vi "mecanum tank 1 sl.vi"   [LabVIEW 2012, in "Mecanum Drive.lvrbt"]
uses:
  Mecanum Drive.lvrbt
  <vilib>/NXT/Hardware/Plugins/Tetrix DC Motor/TetrixDCMotorAddress.ctl
  <vilib>/NXT/NXTIO Xnodes/NXTIONodeSubVIs/TETRIX IO Move DC Motors.vi
  <vilib>/NXT/Dual Mode Library/Display/drawNumber.vi
  <vilib>/NXT/NXTIO Xnodes/NXTIONodeSubVIs/TETRIX IO Check Battery.vi
  <vilib>/NXT/NXTIO Xnodes/NXTIONodeSubVIs/TETRIX IO Stop DC Motors.vi
  <vilib>/NXT/NXTIO Xnodes/AddressXNode/NXTIOAddress.xnode
  <vilib>/NXT/Subs/LVHSConnector.ctl
  <vilib>/NXT/NXTIO Xnodes/NXTIOXNode/NXTIO.xnode
  <vilib>/NXT/LegoClasses/BrickReference/BrickReference.lvclass
panel:
  # "This VI was generated based on your configuration in the Remote Control Editor. You may modify the code as needed for your robot. To test this program for an FTC match, return to the Remote Control Editor, select the \"Run Program\" tab, and choose \"Teleop\"."
types:
  T1 = typedef "TetrixDCMotorAddress.ctl" = i32
  T2 = cluster{"TetrixDCMotor":T1, "TetrixDCMotor 2":T1}
  T3 = typedef "LVHSConnector.ctl" = refnum<class "BrickReference.lvclass">
  T4 = typedef "FTC ControllerState.ctl" = cluster{"Left X":i8, "Left Y":i8, "Right X":i8, "Right Y":i8, "Button Encoding 9-12":u8, "Button Encoding 1-8":u8, "POV":T5}
  T5 = typedef "FTC POVState.ctl" = i8
  T6 = typedef "FTC ButtonEventType.ctl" = enum16{"Pressed", "Released"}
  T7 = cluster{"Button ID":enum16{"None", "Button 1", "Button 2", "Button 3", "Button 4", "Button 5", "Button 6", "Button 7", "Button 8", "Button 9", "Button 10", "Button 11", "Button 12", "POV Up", "POV Up Right", "POV Right", "POV Down Right", "POV Down", "POV Down Left", "POV Left", "POV Up Left"}, "Event Type":T6}[]
  T8 = typedef "FTC ButtonState.ctl" = cluster{"Button 1":bool, "Button 2":bool, "Button 3":bool, "Button 4":bool, "Button 5":bool, "Button 6":bool, "Button 7":bool, "Button 8":bool, "Button 9":bool, "Button 10":bool, "Button 11":bool, "Button 12":bool, "POV":T5}
  T9 = enum16{"None", "Button 1", "Button 2", "Button 3", "Button 4", "Button 5", "Button 6", "Button 7", "Button 8", "Button 9", "Button 10", "Button 11", "Button 12", "POV Up", "POV Up Right", "POV Right", "POV Down Right", "POV Down", "POV Down Left", "POV Left", "POV Up Left"}
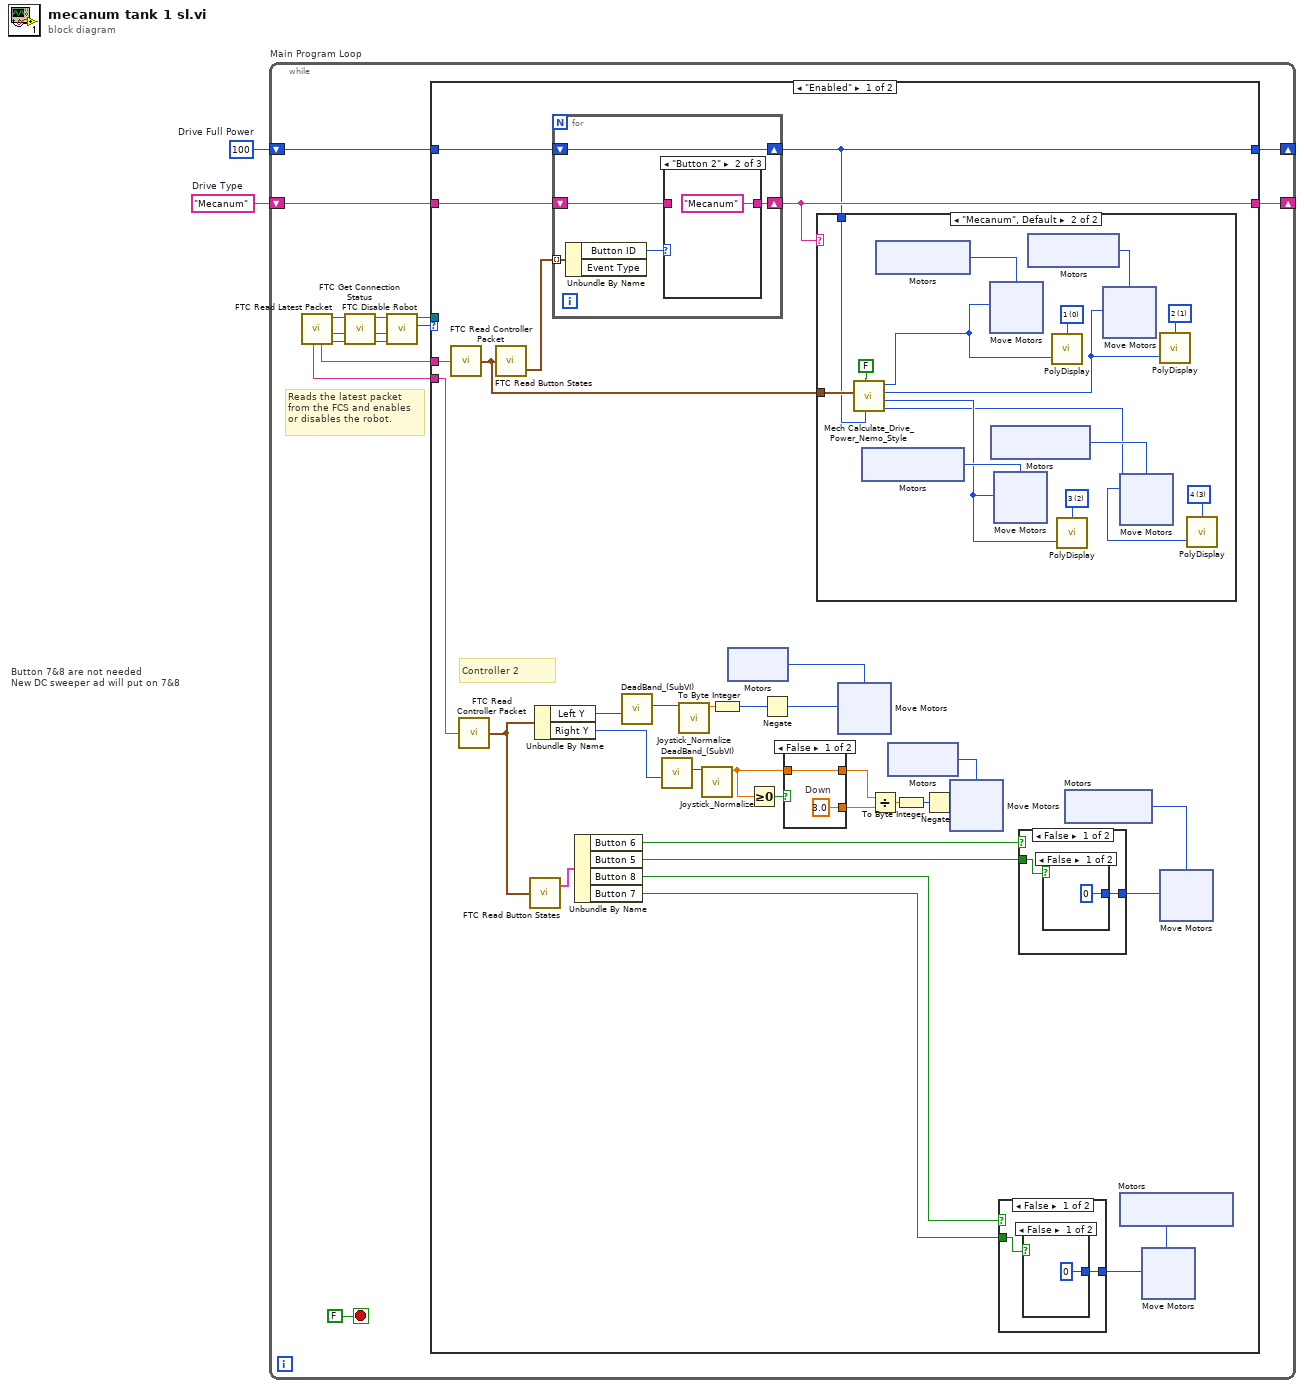
[diagram p0: block diagram]
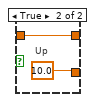
[diagram p2: hidden frame]
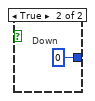
[diagram p3: hidden frame]
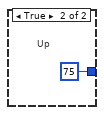
[diagram p4: hidden frame]
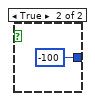
[diagram p5: hidden frame]
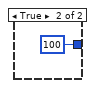
[diagram p6: hidden frame]
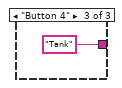
[diagram p9: hidden frame]
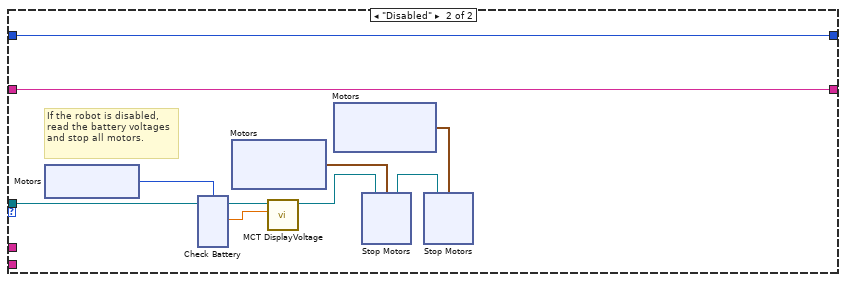
[diagram p10: hidden frame]
diagram:
  w1 = 100  # Drive Full Power
  w2 = "Mecanum"  # Drive Type
  # "Button 7&8 are not needed\nNew DC sweeper ad will put on 7&8"
  n1 = while "Main Program Loop" {
    shift-right: [w5] -> _
    shift-left: w2 -> [w6]
    shift-right: [w3] -> _
    shift-left: w1 -> [w4]
    stop <- FALSE stop-if-true
    # "Reads the latest packet\nfrom the FCS and enables\nor disables the robot."
    n2 = call <vilib>:"FTC Read Latest Packet.vi"() -> ("Packet Received?"=w14:bool, "Stopped?"=w11:bool, "NXT"=w13:T3, "Controller 1"=w16:string, "Controller 2"=w15:string)  [unwired: 6 in, 1 out]
    n3 = call <vilib>:"FTC Get Connection Status.vi"("Packet Received?"=w14, "Stopped?"=w11, "NXT"=w13) -> ("Online?"=w8:bool, "Stopped?"=w9:bool, "NXT"=w10:T3)  [unwired: 5 in]
    n4 = call <vilib>:"FTC Disable Robot.vi"("Online?"=w8, "Stopped?"=w9, "NXT"=w10) -> ("Enabled?"=w12:enum16{"Disabled", "Enabled"}, "NXT"=w7:T3)  [unwired: 3 in]
    n5 = case "disableCase" shown="\"Enabled\"" w12 {
      tunnel: w16 -> [w51 _]
      tunnel: w15 -> [w50 _]
      tunnel: w7 -> [_ w162]
      tunnel: w6 -> [w48 w154]
      tunnel: [w47 w154] -> w5
      tunnel: w4 -> [w45 w153]
      tunnel: [w44 w153] -> w3
      frame "Enabled" {
        # "Controller 2"
        n6 = call <vilib>:"FTC Read Controller Packet.vi"("Packet"=w51) -> ("Controller State"=w46:T4)  [unwired: 4 in]
        n7 = call <vilib>:"FTC Read Controller Packet.vi"("Packet"=w50) -> ("Controller State"=w37:T4)  [unwired: 4 in]
        n8 = call <vilib>:"FTC Read Button States.vi"("Controller State"=w46) -> ("Button Events"=w49:T7)  [unwired: 2 in, 1 out]
        n9 = call <vilib>:"FTC Read Button States.vi"("Controller State"=w37) -> ("Button States"=w36:T8)  [unwired: 2 in, 1 out]
        n10 = Unbundle By Name(w37) -> ("Left Y"=w43:i8, "Right Y"=w38:i8)
        n11 = for {
          tunnel: w49 -> [w149] mode=indexing
          shift-right: [w147] -> w47
          shift-left: w48 -> [w146]
          shift-right: [w145] -> w44
          shift-left: w45 -> [w145]
          n12 = Unbundle By Name(w149) -> ("Button ID"=w148:T9)  [unwired: 1 out]
          n13 = case shown="\"Button 2\"" w148 {
            tunnel: [w150 "Mecanum" "Tank"] -> w147
            tunnel: w146 -> [w150 _ _]
            frame "None", Default {
            }
            frame "Button 2" {
            }
            frame "Button 4" {
            }
          }
        }
        n14 = Unbundle By Name(w36) -> ("Button 6"=w33:bool, "Button 5"=w32:bool, "Button 8"=w28:bool, "Button 7"=w27:bool)
        n15 = call "DeadBand_(SubVI).vi"("Axis In"=w43) -> ("Axis out"=w42:i8)  [unwired: 10 in]
        n16 = call "DeadBand_(SubVI).vi"("Axis In"=w38) -> ("Axis out"=w39:i8)  [unwired: 10 in]
        n17 = call "Joystick_Normalize.vi"("Joystick In"=w42) -> ("Norm Out"=w41:sgl)  [unwired: 10 in]
        n18 = call "Joystick_Normalize.vi"("Joystick In"=w39) -> ("Norm Out"=w21:sgl)  [unwired: 10 in]
        n19 = To Byte Integer(number=w41) -> (8bit integer=w24:i8)
        n20 = xnode "Motors"() -> ("Motor"=w40:T1)
        n21 = Greater Or Equal To 0?(x=w21) -> (x >= 0?=w22:bool)
        n22 = Negate(x=w24) -> (-x=w23:i8)
        n23 = case shown="False" w22 {
          tunnel: [w60 w62] -> w19
          tunnel: w21 -> [w60 w62]
          tunnel: [3.0 10.0] -> w20
          frame False {
            # "Down"
          }
          frame True {
            # "Up"
          }
        }
        n24 = case shown="\"Mecanum\", Default" w47 {
          tunnel: w46 -> [_ w100]
          tunnel: w44 -> [_ w98]
          frame "Tank" {
          }
          frame "Mecanum", Default {
            w102 = i16 3 items=["1", "2", "3", "4", "5", "6", "7", "8", "9", "10", "11", "12"] ("Line")
            w104 = i16 2 items=["1", "2", "3", "4", "5", "6", "7", "8", "9", "10", "11", "12"] ("Line")
            w106 = i16 1 items=["1", "2", "3", "4", "5", "6", "7", "8", "9", "10", "11", "12"] ("Line")
            w107 = i16 0 items=["1", "2", "3", "4", "5", "6", "7", "8", "9", "10", "11", "12"] ("Line")
            n25 = call "Mech Calculate_Drive_Power_Nemo_Style.vi"("Power"=w98, "Reverse"=FALSE, "Controller State"=w100) -> ("Right Rear Power"=w101:i8, "Right Front Power"=w103:i8, "Left Rear Power"=w105:i8, "Left Front Power"=w99:i8)  [unwired: 5 in]
            n26 = xnode ("Motors")() -> ("Motor"=w112:T1)
            n27 = xnode ("Motors")() -> ("Motor"=w109:T1)
            n28 = xnode ("Move Motors")("Power/Speed 1"=w99, "Motors"=w109) -> ()  [unwired: 1 in, 1 out]
            n29 = xnode ("Motors")() -> ("Motor"=w111:T1)
            n30 = xnode ("Move Motors")("Power/Speed 1"=w103, "Motors"=w112) -> ()  [unwired: 1 in, 1 out]
            n31 = xnode ("Motors")() -> ("Motor"=w110:T1)
            n32 = call-poly <vilib>:"PolyDisplay.vi"("number"=w99, "Line"=w107) -> ()  [unwired: 2 in, 1 out]
            n33 = call-poly <vilib>:"PolyDisplay.vi"("number"=w103, "Line"=w104) -> ()  [unwired: 2 in, 1 out]
            n34 = xnode ("Move Motors")("Power/Speed 1"=w105, "Motors"=w110) -> ()  [unwired: 1 in, 1 out]
            n35 = xnode ("Move Motors")("Power/Speed 1"=w101, "Motors"=w111) -> ()  [unwired: 1 in, 1 out]
            n36 = call-poly <vilib>:"PolyDisplay.vi"("number"=w105, "Line"=w106) -> ()  [unwired: 2 in, 1 out]
            n37 = call-poly <vilib>:"PolyDisplay.vi"("number"=w101, "Line"=w102) -> ()  [unwired: 2 in, 1 out]
          }
        }
        n38 = xnode "Move Motors"("Power/Speed 1"=w23, "Motors"=w40) -> ()  [unwired: 1 in, 1 out]
        n39 = Divide(x=w19, y=w20) -> (x/y=w25:dbl)
        n40 = xnode "Motors"() -> ("Motor"=w35:T1)
        n41 = To Byte Integer(number=w25) -> (8bit integer=w34:i8)
        n42 = Negate(x=w34) -> (-x=w26:i8)
        n43 = xnode "Move Motors"("Power/Speed 1"=w26, "Motors"=w35) -> ()  [unwired: 1 in, 1 out]
        n44 = case shown="False" w28 {
          tunnel: w27 -> [w64 _]
          tunnel: [w63 u8 75] -> w18
          frame False {
            n45 = case shown="False" w64 {
              tunnel: [u8 0 u8 0] -> w63
              frame False {
              }
              frame True {
                # "Down"
              }
            }
          }
          frame True {
            # "Up"
          }
        }
        n46 = case shown="False" w33 {
          tunnel: w32 -> [w78 _]
          tunnel: [w77 i8 100] -> w30
          frame False {
            n47 = case shown="False" w78 {
              tunnel: [i8 0 i8 -100] -> w77
              frame False {
              }
              frame True {
              }
            }
          }
          frame True {
          }
        }
        n48 = xnode "Motors"() -> ("Motor"=w31:T1)
        n49 = xnode "Motors"() -> ("Motor"=w29:T1)
        n50 = xnode "Move Motors"("Power/Speed 1"=w18, "Motors"=w29) -> ()  [unwired: 1 in, 1 out]
        n51 = xnode "Move Motors"("Power/Speed 1"=w30, "Motors"=w31) -> ()  [unwired: 1 in, 1 out]
      }
      frame "Disabled" {
        # "If the robot is disabled, read the battery voltages and stop all motors."
        n52 = xnode ("Motors")() -> ("Motor"=w161:T1)
        n53 = xnode ("Check Battery")("Motors"=w161, "NXT/EV3"=w162) -> ("Voltage 1"=w160:sgl, "NXT/EV3"=w159:T3)
        n54 = xnode "Motors"() -> ("Motor"=w158:cluster{"TetrixDCMotor":T1, "TetrixDCMotor":T1})
        n55 = call <vilib>:"MCT DisplayVoltage.vi"("Motor Voltage"=w160, "NXT"=w159) -> ("NXT"=w157:T3)  [unwired: 9 in]
        n56 = xnode "Motors"() -> ("Motor"=w156:cluster{"TetrixDCMotor":T1, "TetrixDCMotor":T1})
        n57 = xnode "Stop Motors"("Motors"=w158, "NXT/EV3"=w157) -> ("NXT/EV3"=w155:T3)
        n58 = xnode "Stop Motors"("Motors"=w156, "NXT/EV3"=w155) -> ()  [unwired: 1 out]
      }
    }
  }
